vi "Map RP Modules.vi"(5 "Modules":i32[](array[numeric]), 6 "Get calibration":bool=TRUE, 7 "Logic tags":u16[](array[numeric])=[101, 102], 8 "Error In":errorcluster, 9 "End address for stand-alone":i32=119, 10 "Subnet":string="192.168.1", 11 "Addresses":string[](array[string])) -> (0 "Error Out":errorcluster, 3 "RP modules map":T1(c390))   [LabVIEW 2024]
uses:
  RP Core/RP Instrument/RP Instrument.lvclass
  <vilib>/Utility/miscctls.llb/LVMapReplaceAction.ctl
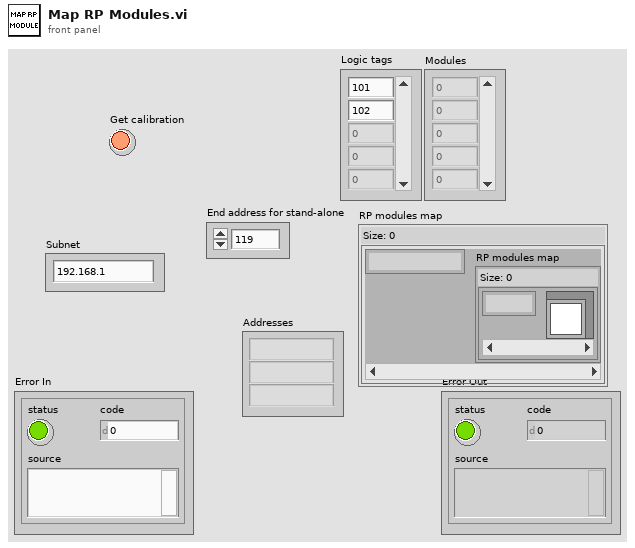
[diagram p1: front panel]
types:
  T1 = map{string, map{i32, refnum<class "RP Instrument.lvclass">}}
  T2 = typedef "LVMapReplaceAction.ctl" = enum32{"Modify Entry only if found", "Add or Modify Entry", "Delete Entry"}
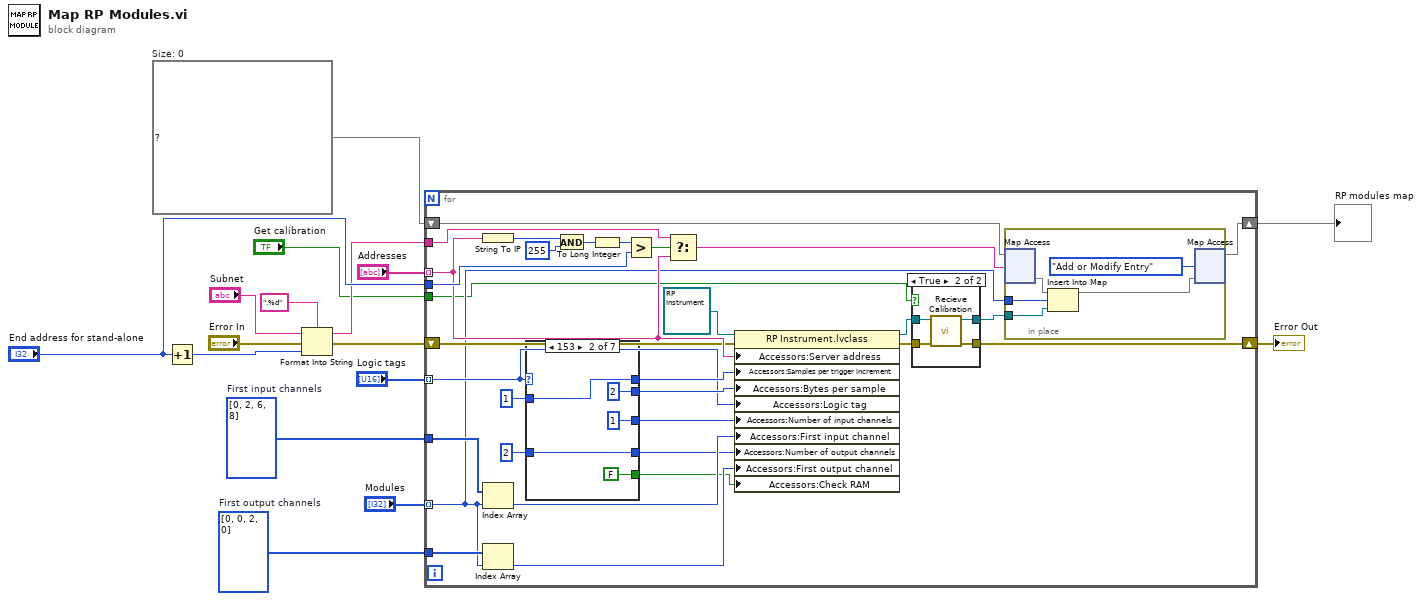
[diagram p0: block diagram]
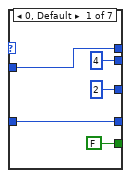
[diagram p3: hidden frame]
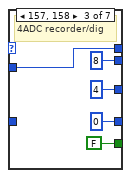
[diagram p4: hidden frame]
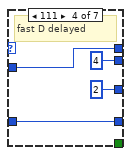
[diagram p5: hidden frame]
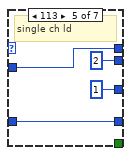
[diagram p6: hidden frame]
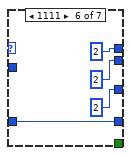
[diagram p7: hidden frame]
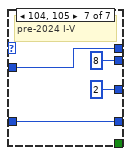
[diagram p8: hidden frame]
diagram:
  w2 = i32[] [0, 0, 2, 0]  # First output channels
  w3 = i32[] [0, 2, 6, 8]  # First input channels
  w16 = T1 {}  # Size: 0
  n1 = Increment(x="End address for stand-alone") -> (x+1=w14:i32)
  n2 = Format Into String(format string=".%d", initial string="Subnet", error in="Error In", w14) -> (resulting string=w8:string, error out=w9:errorcluster)
  n3 = for {
    shift-right: [w33] -> w4
    shift-left: w16 -> [w47]
    tunnel: "Addresses" -> [w38] mode=indexing
    tunnel: "End address for stand-alone" -> [w42]
    tunnel: w8 -> [w40]
    tunnel: "Logic tags" -> [w34] mode=indexing
    tunnel: "Modules" -> [w27] mode=indexing
    shift-right: [w19] -> w15
    shift-left: w9 -> [w32]
    tunnel: w3 -> [w29]
    tunnel: w2 -> [w28]
    tunnel: "Get calibration" -> [w18]
    n4 = String To IP(1:w38) -> (0:w46:u32)
    n5 = Index Array(array=w29, index=w27) -> (element=w30:i32)
    n6 = Index Array(array=w28, index=w27) -> (element=w24:i32)
    n7 = case shown="153" w34 {
      tunnel: [4 ("Trigger granularity") 2 ("Trigger granularity") 8 ("Trigger granularity") 4 ("Trigger granularity") 2 ("Trigger granularity") 2 ("Trigger granularity") 8 ("Trigger granularity")] -> w35
      tunnel: 1 ("Samples per trigger increment") -> [w57 w62 w67 w71 w75 _ w83]
      tunnel: [w57 w62 w67 w71 w75 2 ("Samples per trigger increment") w83] -> w36
      tunnel: [2 ("Trigger granularity") 1 ("Trigger granularity") 4 ("Trigger granularity") 2 ("Trigger granularity") 1 ("Trigger granularity") 2 ("Trigger granularity") 2 ("Trigger granularity")] -> w17
      tunnel: 2 ("Samples per trigger increment") -> [w55 w60 _ w69 w73 w77 w81]
      tunnel: [w55 w60 0 ("Samples per trigger increment") w69 w73 w77 w81] -> w25
      tunnel: [FALSE FALSE FALSE _ _ _ _] -> w23
      frame 0, Default {
      }
      frame 153 {
      }
      frame 157, 158 {
        # "4ADC recorder/dig"
      }
      frame 111 {
        # "fast D delayed"
      }
      frame 113 {
        # "single ch ld"
      }
      frame 1111 {
      }
      frame 104, 105 {
        # "pre-2024 I-V"
      }
    }
    n8 = And(x=w46, y=u32 255) -> (x .and. y?=w45:u32)
    n9 = To Long Integer(number=w45) -> (32bit integer=w43:i32)
    n10 = Greater?(x=w43, y=w42) -> (0:w41:bool)
    n11 = Select(t=w40, s=w41, f=w38) -> (s? t:f=w39:string)
    n12 = property class="RP Instrument.lvclass"(reference=refnum<class "RP Instrument.lvclass"> refnum ("Accessors:RP Instrument"), error in=w32, "Accessors:Server address"=w38, "Accessors:Samples per trigger increment "=w36, "Accessors:Bytes per sample"=w35, "Accessors:Logic tag"=w34, "Accessors:Number of input channels"=w17, "Accessors:First input channel"=w30, "Accessors:Number of output channels"=w25, "Accessors:First output channel"=w24, "Accessors:Check RAM"=w23) -> (reference out=w22:refnum<class "RP Instrument.lvclass">, error out=w20:errorcluster)
    n13 = case shown="True" w18 {
      tunnel: w22 -> [w48 w53]
      tunnel: [w48 w52] -> w21
      tunnel: w20 -> [w49 w51]
      tunnel: [w49 w50] -> w19
      frame False {
      }
      frame True {
        n14 = call-dynamic "Recieve Calibration.vi"("error in (no error)"=w51, "RP Instrument in"=w53) -> ("error out"=w50:errorcluster, "RP Instrument out"=w52:refnum<class "RP Instrument.lvclass">)  [unwired: 7 in, 1 out]
      }
    }
    n15 = in-place {
      in-place-border: w27 -> [w87]
      in-place-border: w21 -> [w86]
      n16 = in-place-map #1(w47, w39) -> (w88:map{i32, refnum<class "RP Instrument.lvclass">})  [unwired: 1 in, 1 out]
      n17 = Insert Into Map(map in=w88, key=w87, value=w86) -> (map out=w85:map{i32, refnum<class "RP Instrument.lvclass">})  [unwired: 2 out]
      n18 = in-place-map #1(w85, LVMapReplaceAction."Add or Modify Entry" ("action")) -> (w33:T1)  [unwired: 2 out]
    }
  }
  "Error Out" <- w15
  "RP modules map" <- w4
